vi "UDP Receive.vi"() -> (0 "Selected Target Info":T1)   [LabVIEW 2011]
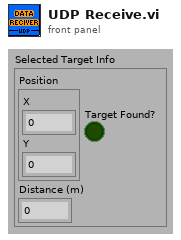
[diagram p1: front panel]
types:
  T1 = cluster{"Position":cluster{"X":dbl, "Y":dbl}, "Distance (m)":dbl, "Target Found?":bool}
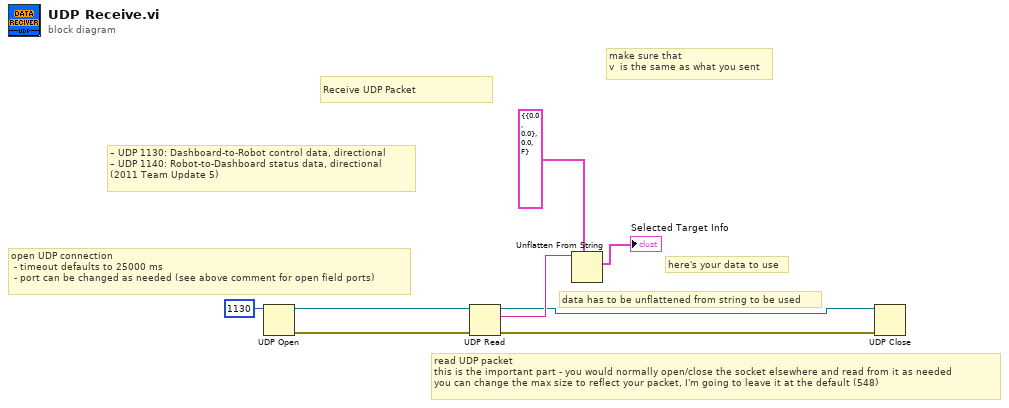
[diagram p0: block diagram]
diagram:
  # "here's your data to use"
  # "make sure that\nv  is the same as what you sent"
  # "data has to be unflattened from string to be used"
  # "read UDP packet\nthis is the important part - you would normally open/close the socket elsewhere and read from it as needed\nyou can change the max size to reflect your packet, I'm going to leave it at the default (548)"
  # "open UDP connection\n - timeout defaults to 25000 ms\n - port can be changed as needed (see above comment for open field ports)"
  # "– UDP 1130: Dashboard-to-Robot control data, directional\n– UDP 1140: Robot-to-Dashboard status data, directional\n(2011 Team Update 5)"
  # "Receive UDP Packet"
  n1 = UDP Open(11:u16 1130 ("port")) -> (port=w7:refnum<k16>, 0:w6:errorcluster)  [unwired: 1 in, 4 out]
  n2 = UDP Read(connection ID=w7, 8:w6) -> (data out=w5:string, error out=w3:errorcluster, 3:w4:refnum<k16>)  [unwired: 4 out]
  n3 = Unflatten From String(type=T1 {"Position"={"X"=0.0, "Y"=0.0}, "Distance (m)"=0.0, "Target Found?"=FALSE} ("Selected Target Info"), binary string=w5) -> (value=→"Selected Target Info":T1)  [unwired: 1 in, 4 out]
  n4 = UDP Close(connection ID=w4, 8:w3) -> ()  [unwired: 2 out]
